vi "1D Array (Normal).vi"(0 "samples":i32=4, 2 "mean":dbl, 4 "std":dbl=1.0, 6 "fixed seed":bool=TRUE, 8 "seed":i32=1729) -> (15 "normal random data":dbl[](array[numeric])=[0.059761770973055295, -1.2840976693409905, 1.1597557331431865, -1.7297253038146831])   [LabVIEW 2014]
uses:
  <vilib>/gmath/statdist.llb/Normal Random.vi
  <vilib>/gmath/NI_Gmath.lvlib
panel:
  out "error":i32
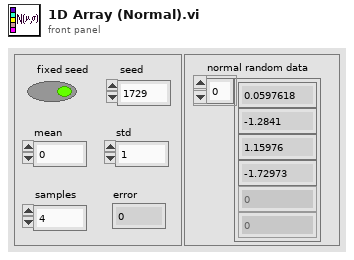
[diagram p1: front panel]
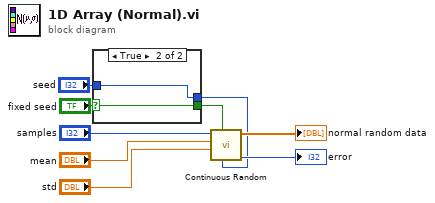
[diagram p0: block diagram]
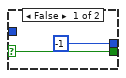
[diagram p2: hidden frame]
diagram:
  n1 = case shown="True" "fixed seed" {
    selector: "fixed seed" -> [w10 w13]
    tunnel: [-1 w12] -> w1
    tunnel: [w10 w13] -> w3
    tunnel: "seed" -> [_ w12]
    frame False {
    }
    frame True {
    }
  }
  n2 = call-poly <vilib>:"Continuous Random.vi"("seed"=w1, "reset"=w3, "std"="std", "mean"="mean", "samples"="samples") -> ("error"=→"error":i32, "normal random data"=→"normal random data":dbl[])  [unwired: 5 in]
